vi "Test.vi"() -> ()   [LabVIEW 2014, in "Generic Power Analyzer.lvlib" / "Generic Power Analyzer.lvclass"]
uses:
  Generic Power Analyzer.lvclass
  <vilib>/ActorFramework/Stop Msg/Stop Msg.lvclass/Stop Msg.ctl
  <vilib>/ActorFramework/Message Enqueuer/Message Enqueuer.lvclass/Message Enqueuer.ctl
  <vilib>/ActorFramework/Message Enqueuer/Enqueue Critical.vi
  <vilib>/ActorFramework/Message Priority Queue/Priority Enqueue.vi
  <vilib>/ActorFramework/Stop Msg/Stop Msg.lvclass
  Generic Instrument/Generic Instrument.lvclass
  <vilib>/ActorFramework/Actor/Actor.lvclass
  SetUp VIs/SetUp VIs.lvlib
panel:
  out "class name":string
  out "Instrument ID":string
  in  "VISA resource name":refnum<visa-resource-name>="USB0::0x0699::0x4002::B010130::INSTR"
  out "error out":errorcluster
  in  "Stop Button":bool
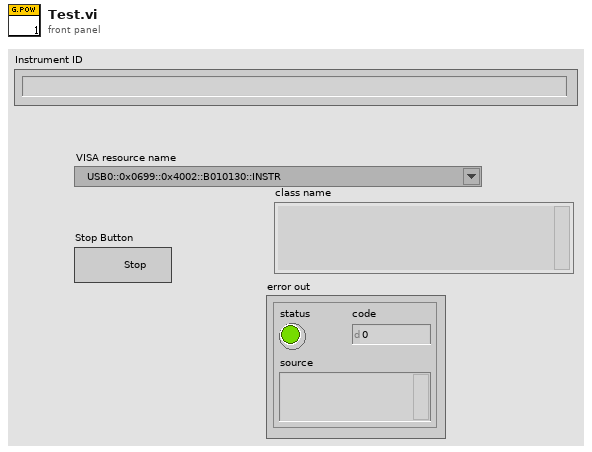
[diagram p1: front panel]
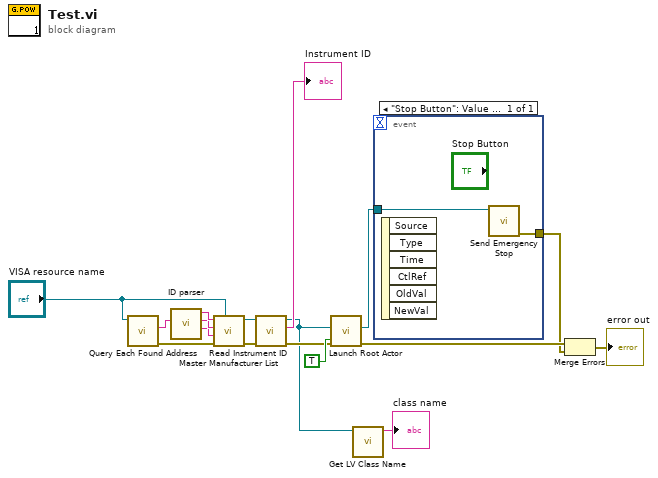
[diagram p0: block diagram]
diagram:
  n1 = call "Query Each Found Address.vi"("Address"="VISA resource name") -> ("error out (no error)"=w8:errorcluster, "read buffer"=w12:string)  [unwired: 9 in]
  n2 = call "ID parser.vi"("Input String"=w12) -> ("Serial"=w9:string, "Model"=w10:string, "Manufacturer"=w11:string)  [unwired: 8 in]
  n3 = call "Master Manufacturer List.vi"("VISA resource name"="VISA resource name", "error in"=w8, "Serial"=w9, "Model"=w10, "Manufacturer"=w11) -> ("error out"=w6:errorcluster, "Generic Instrument out"=w7:refnum<class "Generic Instrument.lvclass">)  [unwired: 5 in]
  n4 = call-dynamic "Read Instrument ID.vi"("error in (no error)"=w6, "Generic Instrument in"=w7) -> ("error out"=w5:errorcluster, "Instrument ID"=→"Instrument ID":string, "Generic Instrument out"=w2:refnum<class "Generic Instrument.lvclass">)  [unwired: 7 in]
  n5 = call <vilib>:"Launch Root Actor.vi"("Open Actor Core front panel? (F)"=TRUE, "error in (no error)"=w5, "Actor"=w2) -> ("error out"=w15:errorcluster, "Actor's Enqueuer"=w16:refnum<class "Message Enqueuer.lvclass">)  [unwired: 7 in]
  n6 = call <vilib>:"Get LV Class Name.vi"("object"=w2) -> ("class name"=→"class name":string)  [unwired: 9 in, 1 out]
  n7 = event shown="[0] \"Stop Button\": Value Change" {
    selector: _ -> [_]
    dyn-events: _ -> [_]
    timeout: _ -> [_]
    tunnel: w16 -> [w19]
    tunnel: [w18] -> w14
    event "Stop Button": Value Change {
      n8 = event-data() -> ()  [unwired: 1 in, 6 out]
      n9 = call <vilib>:"Send Emergency Stop.vi"("Message Enqueuer"=w19) -> ("error out"=w18:errorcluster)  [unwired: 10 in]
    }
  }
  n10 = Merge Errors(w15, w14) -> (→"error out":errorcluster)
